vi "Initialize.vi"(7 "Serial Configuration":cluster{"Baud Rate":u32, "Flow Control":u16}={"Baud Rate"=0, "Flow Control"=4} {"Flow Control" items=["None", "XON/XOFF", "RTS/CTS", "XON/XOFF & RTS/CTS", "DTR/DSR", "XON/XOFF & DTR/DSR"]; "Baud Rate" items=["9600", "19200", "38400", "57600"]}, 8 "error in (no error)":errorcluster {"code" format="%.0x"}, 9 "ID Query (T: Query)":bool=TRUE, 10 "Reset Device (T: Reset)":bool=TRUE, 11 "VISA Resource Name":refnum<visa-resource-name>="GPIB0::7::INSTR") -> (0 "error out":errorcluster {"code" format="%.0x"}, 3 "VISA Resource Name Out":refnum<visa-resource-name>)   [LabVIEW 2011, in "Agilent 546XX Series.lvlib"]
doc: "Passes the addressing information in the instrument resource name to the VISA Open VI and returns the instrument ID.\n\nNote: \nThis instrument driver supports serial communication. If problems are encountered when using serial communication, recommend using baud rates less than 19,200 and hardware handshaking. National Instruments does not provide technical support for the oscilloscope’s physical serial interface. National Instruments will support driver related issues. If you need technical support related to the physical serial interface on either the Agilent 546xx series please contact Agilent"
uses:
  Agilent 546XX Series.lvlib
panel:
  # "© 2003, National Instruments, Corporation.  All Rights Reserved."
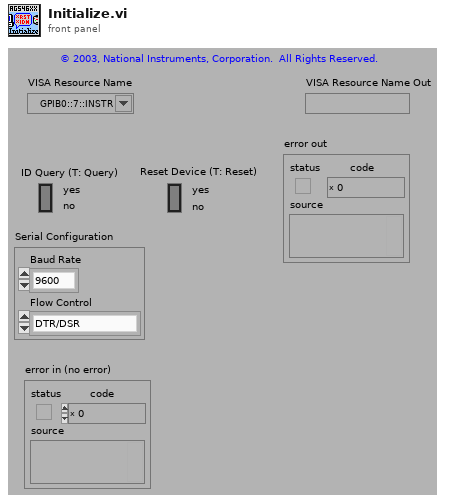
[diagram p1: front panel]
types:
  T1 = cluster{"Status":bool, "Code":i32, "Source (VI Name)":string}
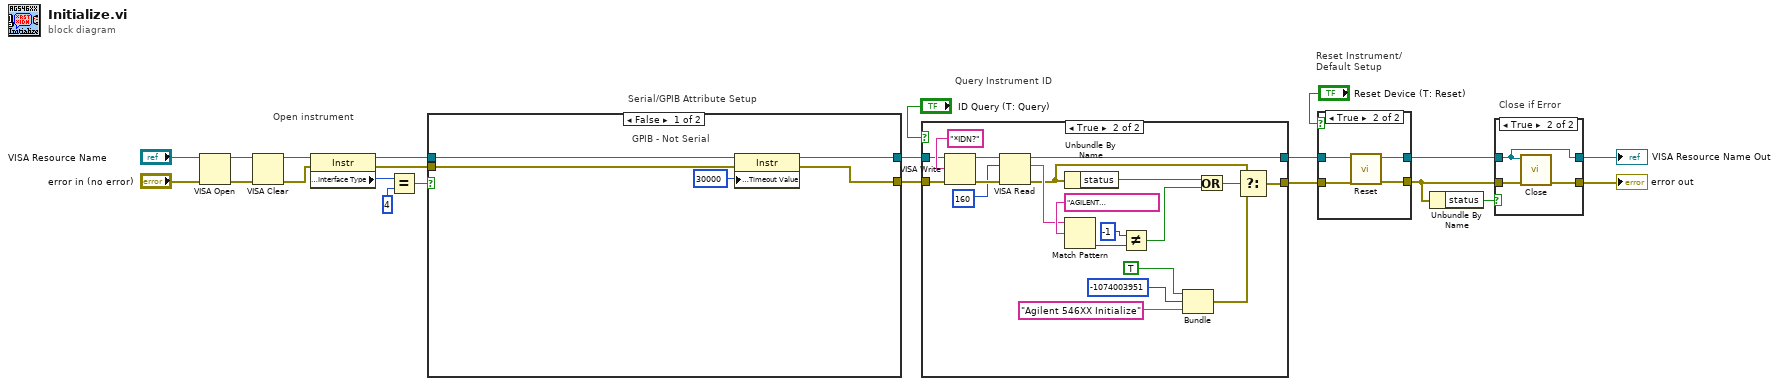
[diagram p0: block diagram]
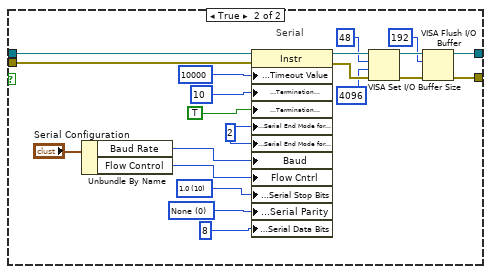
[diagram p3: hidden frame]
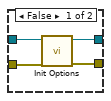
[diagram p5: hidden frame]
diagram:
  # "Serial/GPIB Attribute Setup"
  # "Close if Error"
  # "Reset Instrument/\nDefault Setup"
  # "Open instrument"
  # "Query Instrument ID"
  n1 = VISA Open(error in (no error)="error in (no error)", VISA resource name="VISA Resource Name") -> (VISA resource name=w4:refnum<visa-resource-name>, error out=w3:errorcluster)  [unwired: 3 in]
  n2 = VISA Clear(VISA resource name=w4, error in (no error)=w3) -> (VISA resource name out=w2:refnum<visa-resource-name>, error out=w1:errorcluster)
  n3 = property class="Instr"(reference=w2, error in=w1) -> (reference out=w16:refnum<visa-resource-name>, error out=w17:errorcluster, "Interface Information:Interface Type"=w18:u16)
  n4 = Equal?(x=w18, y=u16 4 ("Serial")) -> (x = y?=w19:bool)
  n5 = case shown="False" w19 {
    tunnel: w16 -> [w27 w40]
    tunnel: w17 -> [w26 w39]
    tunnel: [w25 w38] -> w8
    tunnel: [w24 w37] -> w7
    frame False {
      # "GPIB - Not Serial"
      n6 = property class="Instr"(reference=w27, error in=w26, "General Settings:Timeout Value"=u32 30000) -> (reference out=w25:refnum<visa-resource-name>, error out=w24:errorcluster)
    }
    frame True {
      w35 = u16 0 items=["None", "Odd", "Even", "Mark", "Space"] ("Serial Settings:Serial Parity")
      w36 = u16 10 items=["1.0"=10, "1.5"=15, "2.0"=20] ("Serial Settings:Serial Stop Bits")
      w45 = u16 2 ("ASRL End In")
      # "Serial"
      n7 = Unbundle By Name("Serial Configuration") -> ("Baud Rate"=w29:u32, "Flow Control"=w28:u16)
      n8 = property class="Instr"(reference=w40, error in=w39, "General Settings:Timeout Value"=u32 10000, "Message Based Settings:Termination Character"=u8 10 ("TermChar"), "Message Based Settings:Termination Character Enable"=TRUE ("TermChar En"), "Serial Settings:Serial End Mode for Reads"=w45, "Serial Settings:Serial End Mode for Writes"=w45, "Baud"=w29, "Flow Cntrl"=w28, "Serial Settings:Serial Stop Bits"=w36, "Serial Settings:Serial Parity"=w35, "Serial Settings:Serial Data Bits"=u16 8) -> (reference out=w41:refnum<visa-resource-name>, error out=w42:errorcluster)
      n9 = VISA Set I/O Buffer Size(VISA resource name=w41, mask (16)=u16 48, size (4096)=u32 4096, error in (no error)=w42) -> (VISA resource name out=w44:refnum<visa-resource-name>, error out=w43:errorcluster)
      n10 = VISA Flush I/O Buffer(VISA resource name=w44, mask (16)=u16 192, error in (no error)=w43) -> (VISA resource name out=w38:refnum<visa-resource-name>, error out=w37:errorcluster)
    }
  }
  n11 = case shown="True" "ID Query (T: Query)" {
    tunnel: [w49 w58] -> w12
    tunnel: w7 -> [w49 w62]
    tunnel: [w50 w65] -> w13
    tunnel: w8 -> [w50 w68]
    frame False {
    }
    frame True {
      n12 = VISA Write(VISA resource name=w68, write buffer="*IDN?", error in (no error)=w62) -> (VISA resource name out=w63:refnum<visa-resource-name>, error out=w67:errorcluster)  [unwired: 1 out]
      n13 = VISA Read(VISA resource name=w63, byte count=u32 160, error in (no error)=w67) -> (VISA resource name out=w65:refnum<visa-resource-name>, read buffer=w66:string, error out=w60:errorcluster)  [unwired: 1 out]
      n14 = Unbundle By Name(w60) -> ("status"=w59:bool)
      n15 = Match Pattern(string=w66, regular expression="AGILENT TECHNOLOGIES,546") -> (offset past match=w56:i32)  [unwired: 1 in, 3 out]
      n16 = Not Equal?(x=-1, y=w56) -> (x != y?=w51:bool)
      n17 = Bundle("Status"=TRUE, "Code"=-1074003951, "Source (VI Name)"="Agilent 546XX Initialize") -> (w52:T1)  [unwired: 1 in]
      n18 = Or(x=w59, y=w51) -> (x .or. y?=w61:bool)
      n19 = Select(t=w60, s=w61, f=w52) -> (s? t:f=w58:T1)
    }
  }
  n20 = case shown="True" "Reset Device (T: Reset)" {
    tunnel: w12 -> [w72 w77]
    tunnel: [w73 w75] -> w14
    tunnel: w13 -> [w71 w78]
    tunnel: [w74 w76] -> w15
    frame False {
      n21 = call "Init Options.vi"("error in (no error)"=w72, "VISA Resource Name"=w71) -> ("error out"=w73:errorcluster, "VISA Resource Name Out"=w74:refnum<visa-resource-name>)  [unwired: 8 in]
    }
    frame True {
      n22 = call "Reset.vi"("error in (no error)"=w77, "VISA Resource Name"=w78) -> ("error out"=w75:errorcluster, "VISA Resource Name Out"=w76:refnum<visa-resource-name>)  [unwired: 8 in]
    }
  }
  n23 = Unbundle By Name(w14) -> ("status"=w10:bool)
  n24 = case shown="True" w10 {
    tunnel: w15 -> [w80 w81]
    tunnel: w14 -> [w79 w83]
    tunnel: [w80 w81] -> w6
    tunnel: [w79 w82] -> w5
    frame False {
    }
    frame True {
      n25 = call "Close.vi"("error in (no error)"=w83, "VISA Resource Name"=w81) -> ("error out"=w82:errorcluster)  [unwired: 9 in]
    }
  }
  "error out" <- w5
  "VISA Resource Name Out" <- w6
